vi "READ File.vi"(0 "reference in":refnum<class "RPC.lvclass">, 5 "error in (no error)":errorcluster, 7 "MegaDAC RPC File (*.rsp)":path) -> (14 "reference out":refnum<class "RPC.lvclass">, 19 "error out":errorcluster)   [LabVIEW 2022 SP3, in "RPC.lvclass"]
uses:
  RPC.lvclass
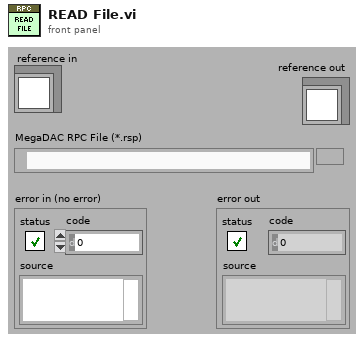
[diagram p1: front panel]
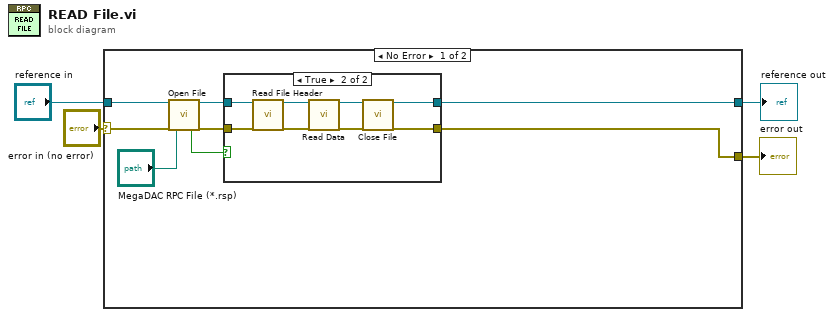
[diagram p0: block diagram]
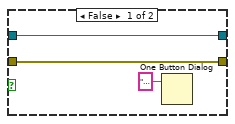
[diagram p2: hidden frame]
diagram:
  n1 = case shown="No Error" "error in (no error)" {
    selector: "error in (no error)" -> [w11 w25]
    tunnel: [w6 w25] -> w3
    tunnel: [w7 w24] -> w1
    tunnel: "reference in" -> [w12 w24]
    frame No Error {
      n2 = call "Open File.vi"("reference in"=w12, "error in (no error)"=w11, "MegaDAC RPC File (*.rsp)"="MegaDAC RPC File (*.rsp)") -> ("file or folder exists?"=w5:bool, "reference out"=w8:refnum<class "RPC.lvclass">, "error out"=w9:errorcluster)  [unwired: 14 in]
      n3 = case shown="True" w5 {
        tunnel: w9 -> [w14 w21]
        tunnel: w8 -> [w15 w20]
        tunnel: [w15 w18] -> w7
        tunnel: [w14 w16] -> w6
        frame False {
          n4 = One Button Dialog(message="Warning, the MegaDAC File (*.rsp) does NOT exist!") -> ()  [unwired: 1 in, 1 out]
        }
        frame True {
          n5 = call "Read File Header.vi"("reference in"=w20, "error in (no error)"=w21) -> ("reference out"=w23:refnum<class "RPC.lvclass">, "error out"=w22:errorcluster)  [unwired: 16 in]
          n6 = call "Read Data.vi"("reference in"=w23, "error in (no error)"=w22) -> ("reference out"=w19:refnum<class "RPC.lvclass">, "error out"=w17:errorcluster)  [unwired: 16 in]
          n7 = call "Close File.vi"("reference in"=w19, "error in (no error)"=w17) -> ("reference out"=w18:refnum<class "RPC.lvclass">, "error out"=w16:errorcluster)  [unwired: 16 in]
        }
      }
    }
    frame Error {
    }
  }
  "error out" <- w3
  "reference out" <- w1
